vi "automatic.vi"(7 "system state in":T1, 11 "mode set":T3) -> (8 "system state out":T1)   [LabVIEW 2016]
doc: "This subvi is responsible to simulate the operations of a normal 4 way intersection, it is a dwell state that it states until is told to leave. Just transition into different states of the intersaction. That includes but not limited to, go, stop, caution, turns, for pedestrians too, and so on.\n\nAlexis Lopez\nP350\nCSUSB Physics"
uses:
  typedefs/control mode enum.ctl
  typedefs/system state cluster.ctl
  typedefs/state enum.ctl
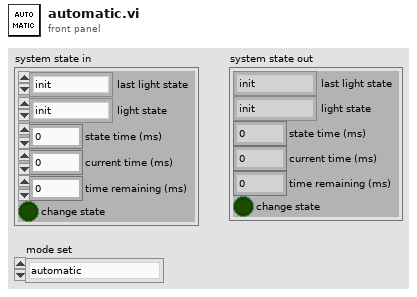
[diagram p1: front panel]
types:
  T1 = typedef "system state cluster.ctl" = cluster{"last light state":T2, "light state":T2, "state time (ms)":i32, "current time (ms)":i32, "time remaining (ms)":i32, "change state":bool}
  T2 = typedef "state enum.ctl" = enum16{"init", "idle", "left turn E", "go EW", "caution EW", "left turn W", "left turn N", "go NS", "caution NS", "left turn S", "blink on", "blink off", "all on test", "exit"}
  T3 = typedef "control mode enum.ctl" = enum16{"automatic", "blinking", "all on test"}
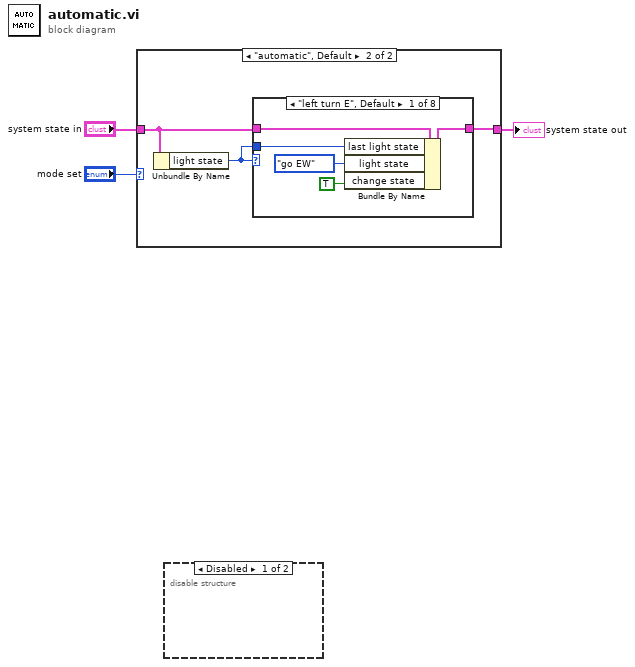
[diagram p0: block diagram]
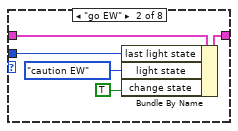
[diagram p3: hidden frame]
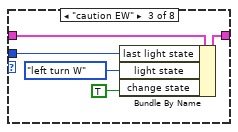
[diagram p4: hidden frame]
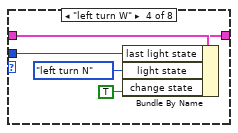
[diagram p5: hidden frame]
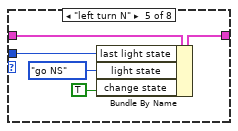
[diagram p6: hidden frame]
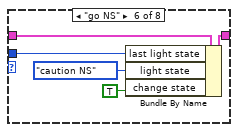
[diagram p7: hidden frame]
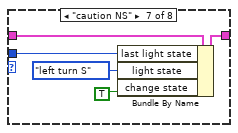
[diagram p8: hidden frame]
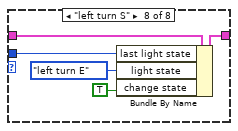
[diagram p9: hidden frame]
diagram:
  n1 = case shown="\"automatic\", Default" "mode set" {
    tunnel: [w4 w7] -> w3
    tunnel: "system state in" -> [w4 w5]
    frame "all on test" {
    }
    frame "automatic", Default {
      n2 = Unbundle By Name(w5) -> ("light state"=w6:T2)
      n3 = case shown="\"left turn E\", Default" w6 {
        tunnel: w5 -> [w12 w17 w22 w27 w32 w37 w42 w47]
        tunnel: [w11 w16 w21 w26 w31 w36 w41 w46] -> w7
        tunnel: w6 -> [w9 w14 w19 w24 w29 w34 w39 w44]
        frame "left turn E", Default {
          n4 = Bundle By Name(cluster=w12, "last light state"=w9, "light state"=state_enum."go EW" ("last light state"), "change state"=TRUE) -> (w11:T1)
        }
        frame "go EW" {
          n5 = Bundle By Name(cluster=w17, "last light state"=w14, "light state"=state_enum."caution EW" ("last light state"), "change state"=TRUE) -> (w16:T1)
        }
        frame "caution EW" {
          n6 = Bundle By Name(cluster=w22, "last light state"=w19, "light state"=state_enum."left turn W" ("last light state"), "change state"=TRUE) -> (w21:T1)
        }
        frame "left turn W" {
          n7 = Bundle By Name(cluster=w27, "last light state"=w24, "light state"=state_enum."left turn N" ("last light state"), "change state"=TRUE) -> (w26:T1)
        }
        frame "left turn N" {
          n8 = Bundle By Name(cluster=w32, "last light state"=w29, "light state"=state_enum."go NS" ("last light state"), "change state"=TRUE) -> (w31:T1)
        }
        frame "go NS" {
          n9 = Bundle By Name(cluster=w37, "last light state"=w34, "light state"=state_enum."caution NS" ("last light state"), "change state"=TRUE) -> (w36:T1)
        }
        frame "caution NS" {
          n10 = Bundle By Name(cluster=w42, "last light state"=w39, "light state"=state_enum."left turn S" ("last light state"), "change state"=TRUE) -> (w41:T1)
        }
        frame "left turn S" {
          n11 = Bundle By Name(cluster=w47, "last light state"=w44, "light state"=state_enum."left turn E" ("last light state"), "change state"=TRUE) -> (w46:T1)
        }
      }
    }
  }
  "system state out" <- w3
  n12 = disable-structure shown="Disabled" {
    frame Disabled {
    }
    frame Enabled {
    }
  }
